vi "SCCSup Get Provider Prefix.vi"(2 "location":string) -> (6 "prefix":string)   [LabVIEW 2020]
doc: "Searches location string for \".llb\" extension. If that is found, the extension is stripped. Otherwise, the value is passed through."
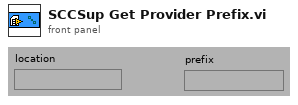
[diagram p1: front panel]
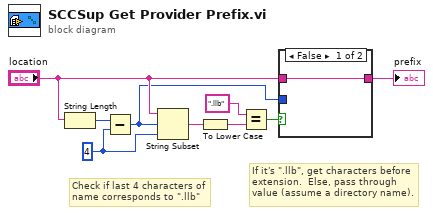
[diagram p0: block diagram]
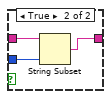
[diagram p2: hidden frame]
diagram:
  w9 = 4
  # "If it's \".llb\", get characters before extension.  Else, pass through value (assume a directory name)."
  # "Check if last 4 characters of name corresponds to \".llb\""
  n1 = String Length(string="location") -> (length=w8:i32)
  n2 = Subtract(x=w8, y=w9) -> (x-y=w1:i32)
  n3 = String Subset(string="location", offset (0)=w1, length (rest)=w9) -> (substring=w7:string)
  n4 = To Lower Case(string=w7) -> (all lower case string=w6:string)
  n5 = Equal?(x=".llb", y=w6) -> (x = y?=w5:bool)
  n6 = case shown="False" w5 {
    tunnel: "location" -> [w10 w13]
    tunnel: [w10 w11] -> w3
    tunnel: w1 -> [_ w12]
    frame False {
    }
    frame True {
      n7 = String Subset(string=w13, length (rest)=w12) -> (substring=w11:string)  [unwired: 1 in]
    }
  }
  "prefix" <- w3
